vi "LibXML_GetContentCastCDATA.vi"(8 "error in":errorcluster, 9 "index":i32, 11 "xmlXPathObj":u32) -> (0 "error out":errorcluster, 2 "content":string="the piezo x axis via adwin analog out", 3 "xmlXPathObj out":u32)   [LabVIEW 2019, in "Tools.lvlib"]
doc: "Gets node content. If CDATA, will handle it appropriately."
uses:
  Tools.lvlib
  libxml2/LibXML_NavigateDirection.ctl
  Error Cluster From Error Code_subroutine.vi
  libxml2/LibXML_GetNodeStrPtr.vi
  libxml2/LibXML_GetNodeResolvedContentStrPointer.vi
  libxml2/LibXML_GetStringLength.vi
  libxml2/LibXML_CopyString.vi
  <vilib>/Utility/error.llb/Trim Whitespace.vi
  LibXML.lvlib
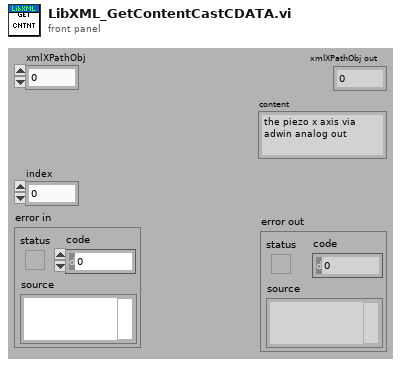
[diagram p1: front panel]
types:
  T1 = typedef "Tools.lvlib/LibXML.lvlib/LibXML_NavigateDirection.ctl" = enum16{"NOP", "first child", "last child", "parent", "next", "prev"}
  T2 = enum16{"nothing", "element", "attribute", "text", "cdata", "5 or more"}
  T3 = enum16{"NOP", "name", "content", "(resolved) content"}
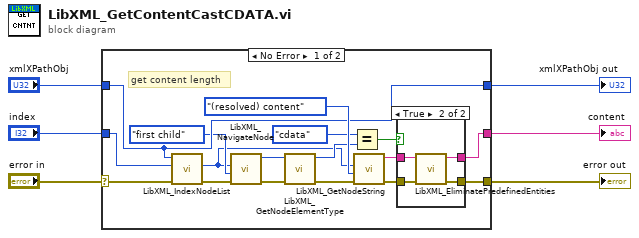
[diagram p0: block diagram]
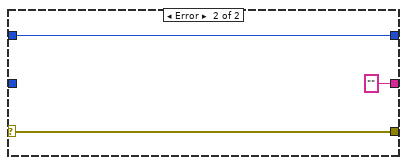
[diagram p3: hidden frame]
diagram:
  n1 = case shown="No Error" "error in" {
    selector: "error in" -> [w23 w32]
    tunnel: [w12 w32] -> w6
    tunnel: [w13 "" ("content")] -> w5
    tunnel: "xmlXPathObj" -> [w16 w30]
    tunnel: [w16 w30] -> w2
    tunnel: "index" -> [w15 _]
    frame No Error {
      # "get content length"
      n2 = call "LibXML_IndexNodeList.vi"("error in"=w23, "index"=w15, "XPathObj"=w16) -> ("error out"=w11:errorcluster, "NodePtr"=w7:u32)  [unwired: 6 in, 1 out]
      n3 = call "LibXML_NavigateNode.vi"("error in (no error)"=w11, "direction"=LibXML_NavigateDirection."first child", "node in"=w7) -> ("error out"=w9:errorcluster, "node out"=w8:u32)  [unwired: 2 in, 1 out]
      n4 = call "LibXML_GetNodeElementType.vi"("error in"=w9, "node"=w8) -> ("error out"=w21:errorcluster, "element type"=w20:T2)  [unwired: 7 in, 1 out]
      n5 = Equal?(x=T2."cdata" ("element type"), y=w20) -> (x = y?=w18:bool)
      n6 = call "LibXML_GetNodeString.vi"("error in"=w21, "type"=T3."(resolved) content", "node"=w7) -> ("error out"=w14:errorcluster, "lvstring"=w17:string)  [unwired: 7 in]
      n7 = case shown="True" w18 {
        tunnel: w17 -> [w24 w26]
        tunnel: w14 -> [w25 w29]
        tunnel: [w24 w28] -> w13
        tunnel: [w25 w27] -> w12
        frame False {
        }
        frame True {
          n8 = call "LibXML_EliminatePredefinedEntities.vi"("error in"=w29, "XML text"=w26) -> ("error out"=w27:errorcluster, "XML (escaped)"=w28:string)  [unwired: 8 in]
        }
      }
    }
    frame Error {
    }
  }
  "error out" <- w6
  "content" <- w5
  "xmlXPathObj out" <- w2
